vi "getName.vi"(8 "error in (no error)":errorcluster, 11 "NullCustomer in":refnum<class "NullCustomer.lvclass">) -> (0 "error out":errorcluster, 2 "name":string, 3 "NullCustomer out":refnum<class "NullCustomer.lvclass">)   [LabVIEW 2017, in "NullCustomer.lvclass"]
uses:
  NullCustomer.lvclass
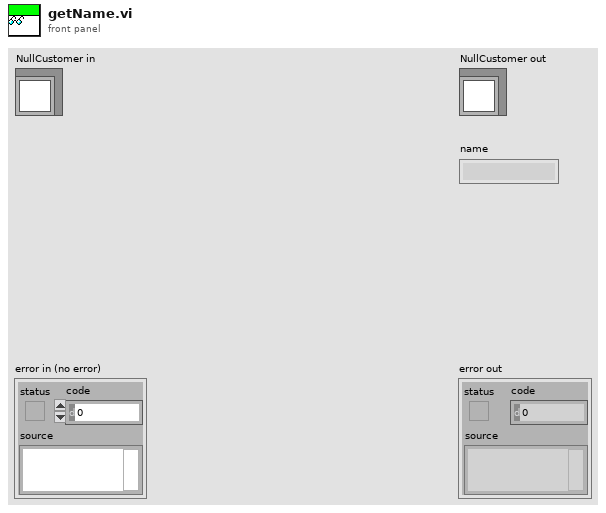
[diagram p1: front panel]
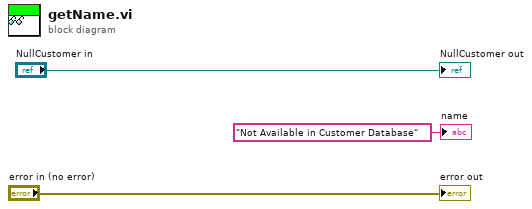
[diagram p0: block diagram]
diagram:
  "error out" <- "error in (no error)"
  "NullCustomer out" <- "NullCustomer in"
  "name" <- "Not Available in Customer Database" ("name")
